vi "Pause Work.vi"(8 "error in (no error)":errorcluster, 11 "Process Controller in":refnum<class "Process Controller.lvclass">) -> (0 "error out":errorcluster, 3 "Process Controller out":refnum<class "Process Controller.lvclass">)   [LabVIEW 2016, in "Process Controller.lvclass"]
uses:
  Process Controller.lvclass
  C:/github/LabActor/Worker/Worker.lvclass
  Worker/Worker State.ctl
  Worker/Worker.lvclass/Worker.ctl
  Worker/Write Pause requested.vi
  Template Module/Read State.vi
  Worker/Read Paused.vi
  Worker/Read Pause requested.vi
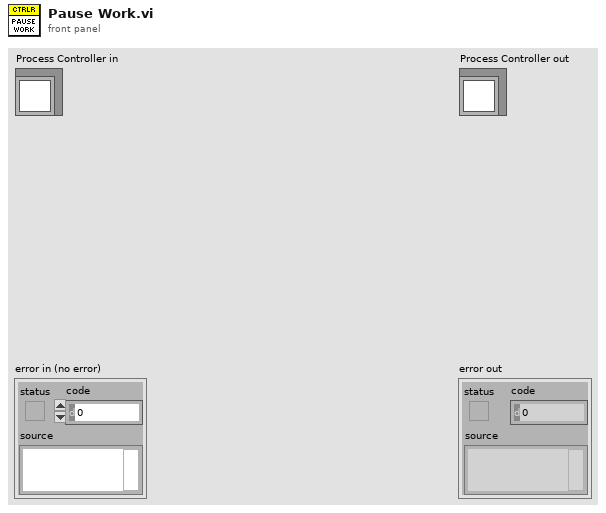
[diagram p1: front panel]
types:
  T1 = typedef "Worker State.ctl" = enum16{"Idle", "Starting", "Working", "Stopping"}
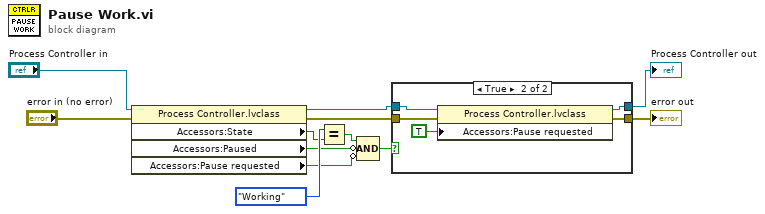
[diagram p0: block diagram]
diagram:
  n1 = property class="Process Controller.lvclass"(reference="Process Controller in", error in="error in (no error)") -> (reference out=w5:refnum<class "Process Controller.lvclass">, error out=w3:errorcluster, "Accessors:State"=w9:T1, "Accessors:Paused"=w8:bool, "Accessors:Pause requested"=w4:bool)
  n2 = Equal?(x=Worker_State."Working" ("State"), y=w9) -> (x = y?=w7:bool)
  n3 = Compound Arithmetic op=AND(w7, invert w8, invert w4) -> (w6:bool)
  n4 = case shown="True" w6 {
    tunnel: w5 -> [w14 w19]
    tunnel: w3 -> [w13 w18]
    tunnel: [w13 w16] -> w2
    tunnel: [w14 w15] -> w1
    frame False {
    }
    frame True {
      n5 = property class="Process Controller.lvclass"(reference=w19, error in=w18, "Accessors:Pause requested"=TRUE ("Pause requested")) -> (reference out=w15:refnum<class "Process Controller.lvclass">, error out=w16:errorcluster)
    }
  }
  "error out" <- w2
  "Process Controller out" <- w1
